vi "getPhaseMeasurement.vi"(8 "error in (no error)":errorcluster, 9 "Source 2":string, 10 "Source 1":string, 11 "ScopeNi in":refnum<class "ScopeNi.lvclass">) -> (0 "error out":errorcluster, 2 "Numeric":dbl, 3 "ScopeNi out":refnum<class "ScopeNi.lvclass">)   [LabVIEW 2023, in "ScopeNi.lvclass"]
doc: "<b>Author:</b> Wolfgang\n<b>Descritpion:</b> Measure the phase shift between two sources."
uses:
  ScopeNi.lvclass
  <instrlib>/niScope/Controls/niScope scalar measurement.ctl
  ScopeNi.lvclass/ScopeNi.ctl
  <instrlib>/niScope/Measurements/niScope Fetch Measurement.vi
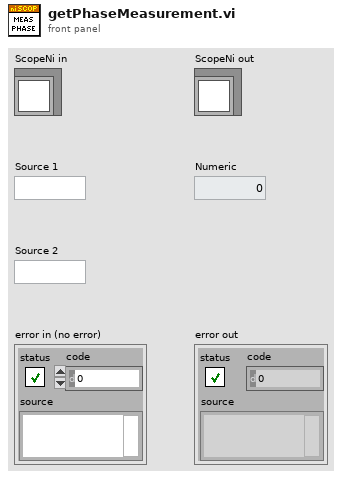
[diagram p1: front panel]
types:
  T1 = typedef "niScope scalar measurement.ctl" = i32
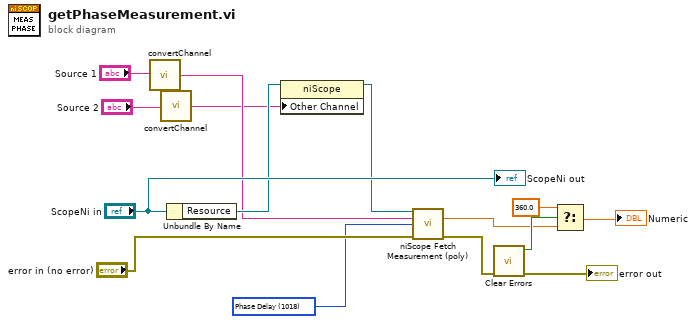
[diagram p0: block diagram]
diagram:
  w6 = T1 1018 items=["None"=4000, "Frequency"=2, "Average Frequency"=1016, "FFT Frequency"=1008, "Period"=3, "Average Period"=1015, "Rise Time"=0, "Fall Time"=1, "Rising Slew Rate"=1010, "Falling Slew Rate"=1011, "Overshoot"=18, "Preshoot"=19, "Voltage RMS"=4, "Voltage Cycle RMS"=16, "AC Estimate"=1012, "FFT Amplitude"=1009, "Voltage Average"=10, "Voltage Cycle Average"=17, "DC Estimate"=1013, "Voltage Max"=6, "Voltage Min"=7, "Voltage Peak-to-Peak"=5, "Voltage High"=8, "Voltage Low"=9, "Voltage Amplitude"=15, "Voltage Top"=1007, "Voltage Base"=1006, "Voltage Base-to-Top"=1017, "Negative Width"=11, "Positive Width"=12, "Negative Duty Cycle"=13, "Positive Duty Cycle"=14, "Integral"=1005, "Area"=1003, "Cycle Area"=1004, "Time Delay"=1014, "Phase Delay"=1018, "Low Ref Volts"=1000, "Mid Ref Volts"=1001, "High Ref Volts"=1002, "Volt. Hist. Mean"=2000, "Volt. Hist. Stdev"=2001, "Volt. Hist. Median"=2003, "Volt. Hist. Mode"=2010, "Volt. Hist. Max"=2005, "Volt. Hist. Min"=2006, "Volt. Hist. Peak-to-Peak"=2002, "Volt. Hist. Mean + Stdev"=2007, "Volt. Hist. Mean + 2 Stdev"=2008, "Volt. Hist. Mean + 3 Stdev"=2009, "Volt. Hist. Hits"=2004, "Volt. Hist. New Hits"=2011, "Time Hist. Mean"=3000, "Time Hist. Stdev"=3001, "Time Hist. Median"=3003, "Time Hist. Mode"=3010, "Time Hist. Max"=3005, "Time Hist. Min"=3006, "Time Hist. Peak-to-Peak"=3002, "Time Hist. Mean + Stdev"=3007, "Time Hist. Mean + 2 Stdev"=3008, "Time Hist. Mean + 3 Stdev"=3009, "Time Hist. Hits"=3004, "Time Hist. New Hits"=3011] ("scalar measurement")
  n1 = call "convertChannel.vi"("Chn in"="Source 1") -> ("Chn out"=w9:string)
  n2 = call "convertChannel.vi"("Chn in"="Source 2") -> ("Chn out"=w8:string)
  n3 = Unbundle By Name("ScopeNi in") -> ("Resource"=w10:refnum<k15>)
  n4 = property class="niScope"(reference=w10, "Other Channel"=w8) -> (reference out=w7:refnum<k15>)  [unwired: 1 in, 1 out]
  n5 = call-poly <instrlib>:"niScope Fetch Measurement (poly).vi"("instrument handle"=w7, "channels"=w9, "scalar measurement"=w6, "error in"="error in (no error)") -> ("result"=w3:dbl, "error out"=w11:errorcluster)  [unwired: 9 in, 1 out]
  n6 = call <vilib>:"Clear Errors.vi"("error in (no error)"=w11) -> ("error out"=→"error out":errorcluster, "specific error cleared?"=w4:bool)  [unwired: 5 in]
  n7 = Select(t=360.0, s=w4, f=w3) -> (s? t:f=→"Numeric":dbl)
  "ScopeNi out" <- "ScopeNi in"
